vi "getCurrentPath.vi"(8 "error in (no error)":errorcluster, 11 "settingsViewer.lvclass in":refnum<class "settingsViewer.lvclass">) -> (0 "error out":errorcluster, 2 "Current Path":path=path "D:/Data/Labview/BEC Suite/Hal/Channels/Camera/XML Camera Settings/CameraSettings.xml", 3 "settingsViewer.lvclass out":refnum<class "settingsViewer.lvclass">)   [LabVIEW 2009, in "Views.lvlib" / "SettingsViewer.lvclass"]
uses:
  settingsViewer.lvclass
  settingsViewer.lvclass/settingsViewer.ctl
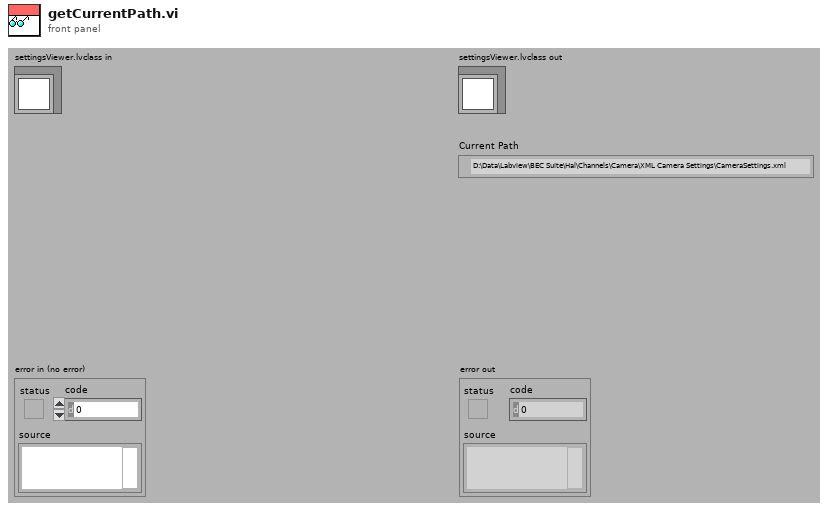
[diagram p1: front panel]
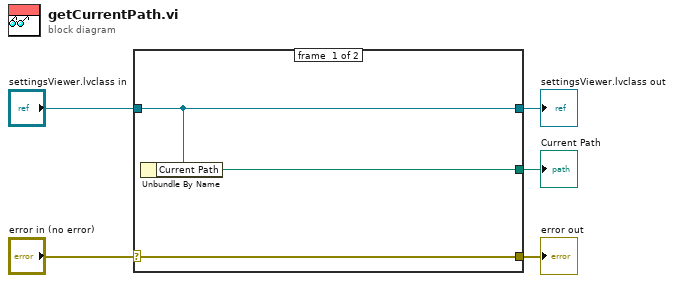
[diagram p0: block diagram]
diagram:
  n1 = case shown="No Error" "error in (no error)" {
    selector: "error in (no error)" -> [w8 w9]
    tunnel: [w8 w9] -> w4
    tunnel: [w7 w10] -> w2
    tunnel: "settingsViewer.lvclass in" -> [w7 w10]
    tunnel: [w6 _] -> w1
    frame #0 {
      n2 = Unbundle By Name(w7) -> ("Current Path"=w6:path)
    }
    frame #1 {
    }
  }
  "error out" <- w4
  "settingsViewer.lvclass out" <- w2
  "Current Path" <- w1
